vi "Acquire.vi"(8 "error in (no error)":errorcluster, 10 "presamp":dbl, 11 "hDevice in":u32) -> (0 "error out":errorcluster, 1 "Stopped?":bool, 2 "Data Out":dbl[][](array[numeric]), 3 "hDevice out":u32)   [LabVIEW 2018]
uses:
  LibTiePie.lvlib
panel:
  out "ScpStarted":bool
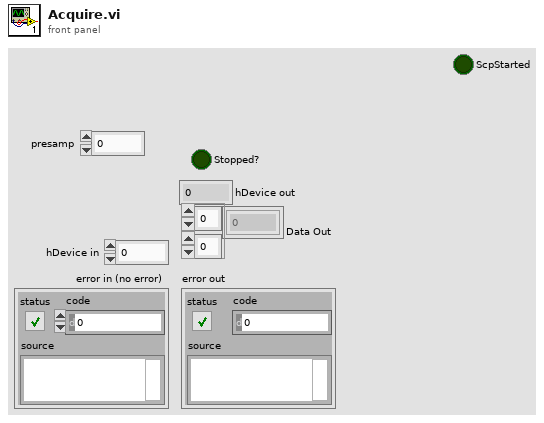
[diagram p1: front panel]
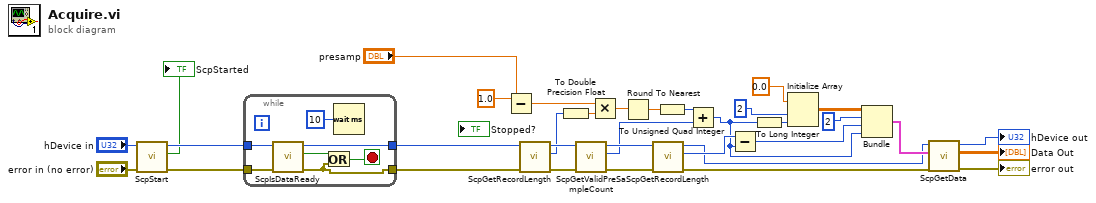
[diagram p0: block diagram]
diagram:
  n1 = call "ScpStart.vi"("error in (no error)"="error in (no error)", "hDevice in"="hDevice in") -> ("error out"=w5:errorcluster, "ScpStarted"=→"ScpStarted":bool, "hDevice out"=w6:u32)  [unwired: 7 in]
  n2 = while {
    tunnel: w6 -> [w41]
    tunnel: w5 -> [w40]
    tunnel: [w35] -> w1
    tunnel: [w38] -> w2
    stop <- w37 stop-if-true
    n3 = call "ScpIsDataReady.vi"("error in (no error)"=w40, "hDevice in"=w41) -> ("error out"=w35:errorcluster, "Data ready?"=w36:bool, "hDevice out"=w38:u32)  [unwired: 7 in]
    n4 = Or(x=w36, y=w35) -> (x .or. y?=w37:bool)
    n5 = Wait (ms)(milliseconds to wait=u32 10) -> ()  [unwired: 1 out]
  }
  n6 = Subtract(x=1.0, y="presamp") -> (x-y=w31:dbl)
  n7 = call "ScpGetRecordLength.vi"("error in (no error)"=w1, "hDevice in"=w2) -> ("error out"=w34:errorcluster, "u64RecordLength"=w29:u64, "hDevice out"=w33:u32)  [unwired: 7 in]
  n8 = To Double Precision Float(number=w29) -> (double precision float=w30:dbl)
  n9 = call "ScpGetValidPreSampleCount.vi"("error in (no error)"=w34, "hDevice in"=w33) -> ("error out"=w25:errorcluster, "dValidPreSampleCount"=w19:u64, "hDevice out"=w24:u32)  [unwired: 7 in]
  n10 = Multiply(x=w31, y=w30) -> (x*y=w28:dbl)
  n11 = Round To Nearest(number=w28) -> (nearest integer value=w27:dbl)
  n12 = call "ScpGetRecordLength.vi"("error in (no error)"=w25, "hDevice in"=w24) -> ("error out"=w12:errorcluster, "u64RecordLength"=w20:u64, "hDevice out"=w13:u32)  [unwired: 7 in]
  n13 = To Unsigned Quad Integer(1:w27) -> (0:w26:u64)
  n14 = Add(x=w26, y=w19) -> (x+y=w15:u64)
  n15 = Subtract(x=w20, y=w15) -> (x-y=w16:u64)
  n16 = To Long Integer(number=w15) -> (32bit integer=w23:i32)
  n17 = Initialize Array(0.0 ("element"), 2 ("dimension size"), w23) -> (w18:dbl[][])
  n18 = Bundle(w18, u16 2, w16, w15) -> (w14:cluster{dbl[][], u16, u64, u64})  [unwired: 1 in]
  n19 = call "ScpGetData.vi"("error in (no error)"=w12, "GetDataCluster"=w14, "hDevice in"=w13) -> ("error out"=→"error out":errorcluster, "Data Out"=→"Data Out":dbl[][], "hDevice out"=→"hDevice out":u32)  [unwired: 5 in, 1 out]
